vi "Spectrum Emission Test.vi"(8 "error in":errorcluster, 9 "Execute":bool, 10 "data":variant) -> (0 "error out":errorcluster)   [LabVIEW 2018, in "LED Control Module.lvlib"]
uses:
  LED Control Module.lvlib
  Private Controls/Module Data Cluster.ctl
  Private Controls/Module Action.ctl
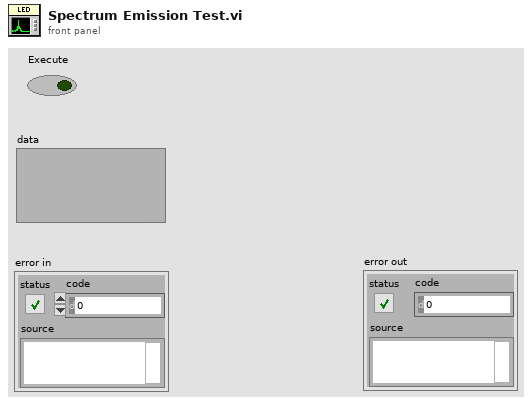
[diagram p1: front panel]
types:
  T1 = typedef "LED Control Module.lvlib/Module Data Cluster.ctl" = cluster{"Variant":variant, "action":T2}
  T2 = typedef "LED Control Module.lvlib/Module Action.ctl" = enum16{"init", "start", "Current", "Spectrum", "WriteResult", "---WIP---", "clear", "error", "close", "exit"}
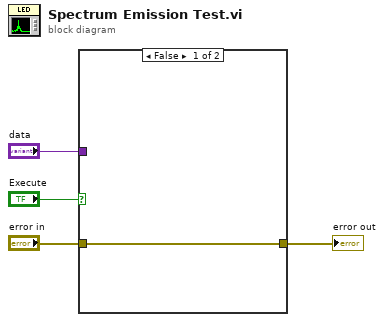
[diagram p0: block diagram]
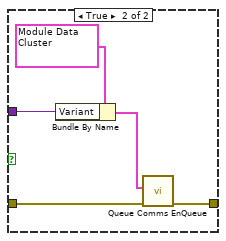
[diagram p2: hidden frame]
diagram:
  n1 = case shown="False" "Execute" {
    tunnel: "error in" -> [w5 w10]
    tunnel: [w5 w9] -> w3
    tunnel: "data" -> [_ w6]
    frame False {
    }
    frame True {
      n2 = Bundle By Name(cluster=T1 {"Variant"=variant, "action"=enum."Spectrum"} ("Module Data Cluster"), "Variant"=w6) -> (w8:T1)
      n3 = call "Queue Comms EnQueue.vi"("error in"=w10, "Module Data Cluster"=w8) -> ("error out"=w9:errorcluster)  [unwired: 9 in]
    }
  }
  "error out" <- w3
